vi "PID_module.vi"() -> ()   [LabVIEW 2020]
uses:
  Testing/Set Time.vi
  <vilib>/addons/control/pid/pid.llb/PID (DBL).vi
  Global Variables/Global Difficulty Level.vi
  <vilib>/addons/control/pid/NI_PID_pid.lvlib
panel:
  out "PID History Graph":dbl(graph)
  in  "PID gains":T1={"proportional gain (Kc)"=1.0, "integral time (Ti, min)"=0.01, "derivative time (Td, min)"=0.0} {"derivative time (Td, min)" format="%.3f"; "integral time (Ti, min)" format="%.3f"; "proportional gain (Kc)" format="%.3f"}
  out "PID Out":dbl
  out "Response ANN":dbl[](array[numeric])
  out "ANN Classification Input":dbl[](array[numeric])
  out "Difficulty Level":u8
  # "These parameters have not been optimized,\nfuture work."
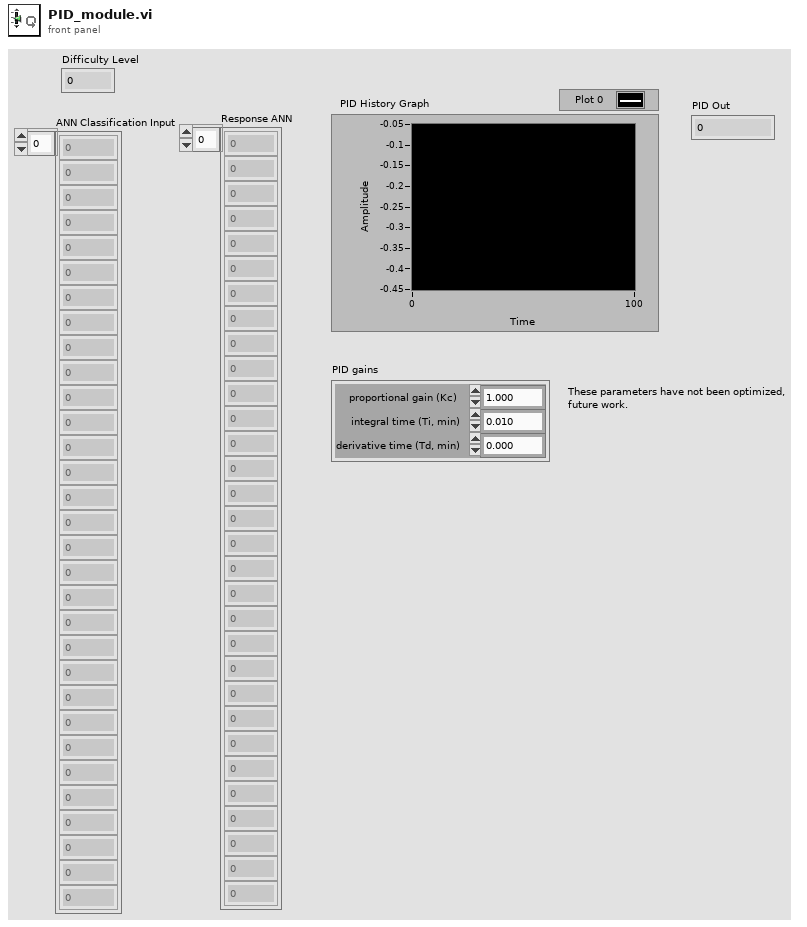
[diagram p1: front panel]
types:
  T1 = cluster{"proportional gain (Kc)":dbl, "integral time (Ti, min)":dbl, "derivative time (Td, min)":dbl}
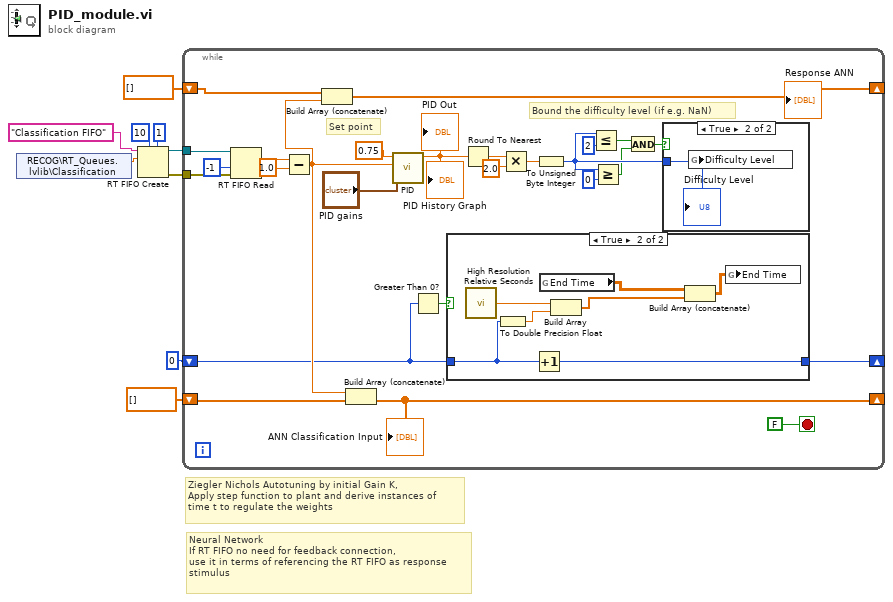
[diagram p0: block diagram]
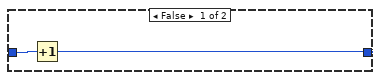
[diagram p3: hidden frame]
diagram:
  # "Neural Network\nIf RT FIFO no need for feedback connection, \nuse it in terms of referencing the RT FIFO as response \nstimulus"
  # "Ziegler Nichols Autotuning by initial Gain K, \nApply step function to plant and derive instances of \ntime t to regulate the weights"
  n1 = shared-variable "RECOG\\RT_Queues.lvlib\\Classification"() -> (w9:dbl)  [unwired: 1 in, 1 out]
  n2 = RT FIFO Create(0:"Classification FIFO" ("name (unnamed)"), 1:w9, 4:u32 10 ("size (10)"), 6:u32 1 ("elements in array (1)")) -> (8:w5:refnum<k33>, 11:w4:errorcluster)  [unwired: 4 in, 1 out]
  n3 = while {
    tunnel: w5 -> [w33]
    tunnel: w4 -> [w34]
    shift-right: [w16] -> _
    shift-left: dbl[] [] -> [w26]
    shift-right: [w25] -> _
    shift-left: dbl[] [] -> [w24]
    shift-right: [w23] -> _
    shift-left: 0 -> [w10]
    stop <- FALSE stop-if-true
    # "Bound the difficulty level (if e.g. NaN)"
    # "Set point"
    n4 = RT FIFO Read(0:w33, 2:-1 ("timeout in ms (0)"), 3:w34) -> (9:w32:dbl)  [unwired: 1 in, 4 out]
    n5 = Subtract(x=w32, y=1.0) -> (x-y=w14:dbl)
    n6 = Build Array (concatenate)(w26, w14) -> (w16:dbl[])
    "Response ANN" <- w16
    n7 = Build Array (concatenate)(w14, w24) -> (w25:dbl[])
    "ANN Classification Input" <- w25
    n8 = call-poly <vilib>:"PID.vi"("PID gains"="PID gains", "process variable"=w14, "setpoint"=0.75) -> ("output"=w12:dbl)  [unwired: 7 in, 1 out]
    "PID Out" <- w12
    "PID History Graph" <- w12
    n9 = Greater Than 0?(x=w10) -> (x > 0?=w11:bool)
    n10 = case shown="True" w11 {
      tunnel: [w37 w39] -> w23
      tunnel: w10 -> [w38 w40]
      frame False {
        n11 = Increment(x=w38) -> (x+1=w37:i32)
      }
      frame True {
        n12 = call <vilib>:"High Resolution Relative Seconds.vi"() -> ("relative seconds"=w45:dbl)
        n13 = To Double Precision Float(number=w40) -> (double precision float=w44:dbl)
        n14 = Increment(x=w40) -> (x+1=w39:i32)
        n15 = global read "Set Time.vi" "End Time"() -> (w41:dbl[][])
        n16 = Build Array(w45, w44) -> (w43:dbl[])
        n17 = Build Array (concatenate)(w41, w43) -> (w42:dbl[][])
        n18 = global write "Set Time.vi" "End Time"(w42) -> ()
      }
    }
    n19 = Round To Nearest(number=w12) -> (nearest integer value=w29:dbl)
    n20 = Multiply(x=w29, y=2.0) -> (x*y=w30:dbl)
    n21 = To Unsigned Byte Integer(number=w30) -> (unsigned 8bit integer=w21:u8)
    n22 = Less Or Equal?(x=w21, y=u8 2) -> (x <= y?=w18:bool)
    n23 = Greater Or Equal?(x=w21, y=u8 0) -> (x >= y?=w17:bool)
    n24 = And(x=w18, y=w17) -> (x .and. y?=w19:bool)
    n25 = case shown="True" w19 {
      tunnel: w21 -> [_ w36]
      frame False {
      }
      frame True {
        n26 = global write "Global Difficulty Level.vi" "Difficulty Level"(w36) -> ()
        "Difficulty Level" <- w36
      }
    }
  }
